vi "New.vi"(8 "error in (no error)":errorcluster, 10 "Parent":refnum<class "Config Element.lvclass">, 11 "Name":string) -> (0 "error out":errorcluster, 3 "SensorList out":refnum<class "SensorList.lvclass">)   [LabVIEW 2020, in "VolatusConfig.lvlib" / "SensorList.lvclass"]
uses:
  SensorList.lvclass
  C:/dev/lv20CE/relink/lv-volatus/VolatusConfig/VolatusConfigElement/VolatusConfigElement.lvclass
  lv-cdm/CDM-Config/Config Element/Config Element.lvclass
  lv-cdm/CDM-Config/Value Type.ctl
  Meta Type.ctl
  Overlays.ctl
  lv-cdm/CDM-Config/CDM-Config.lvlib
  VolatusConfig.lvlib
  VolatusConfigElement/VolatusConfigElement.lvclass
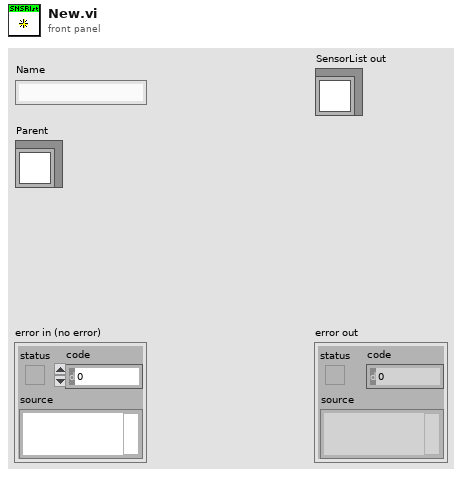
[diagram p1: front panel]
types:
  T1 = typedef "VolatusConfig.lvlib/Overlays.ctl" = enum16{"Sensors", "Wiring"}
  T2 = typedef "VolatusConfig.lvlib/Meta Type.ctl" = enum16{"UNKNOWN", "VL_System", "VL_Cluster", "VL_Node", "VL_Task", "VL_Group", "VL_Channel", "VL_Task_List", "VL_Scaling", "VL_Sensor", "VL_Sensor_List", "VL_Scale"}
  T3 = typedef "CDM-Config.lvlib/Value Type.ctl" = enum16{"String", "Number", "Bool", "Object", "Array"}
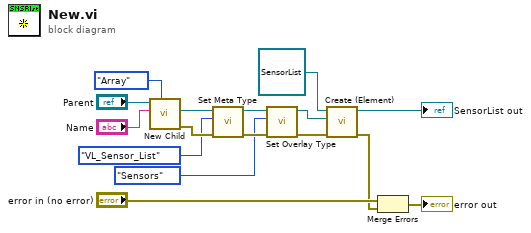
[diagram p0: block diagram]
diagram:
  n1 = call "New Child.vi"("Value Type (String)"=Value_Type."Array", "Child Name"="Name", "Config Element in"="Parent") -> ("error out"=w15:errorcluster, "New Child"=w10:refnum<class "Config Element.lvclass">)  [unwired: 6 in, 1 out]
  n2 = call "Set Meta Type.vi"("error in (no error)"=w15, "Meta Type"=Meta_Type."VL_Sensor_List", "Element In"=w10) -> ("error out"=w16:errorcluster, "Element"=w8:refnum<class "Config Element.lvclass">)  [unwired: 7 in]
  n3 = call "Set Overlay Type.vi"("error in (no error)"=w16, "Overlay Type"=Overlays."Sensors", "Element In"=w8) -> ("error out"=w6:errorcluster, "Element"=w5:refnum<class "Config Element.lvclass">)  [unwired: 7 in]
  n4 = call "Create (Element).vi"("error in (no error)"=w6, "Element"=w5, "VolatusConfigElement in"=refnum<class "SensorList.lvclass"> refnum ("SensorList in")) -> ("error out"=w1:errorcluster, "VolatusConfigElement out"=→"SensorList out":refnum<class "SensorList.lvclass">)  [unwired: 7 in]
  n5 = Merge Errors("error in (no error)", w1) -> (→"error out":errorcluster)
